vi "Edited-PumpCMD&Query(SubVI).vi"(0 "VISA资源名称":refnum<visa-resource-name>, 1 "允许执行时间":u32, 5 "命令":string, 7 "急停":string, 9 "查询":string, 11 "错误输入（无错误）":errorcluster, 12 "emergence":refnum<vi>) -> (4 "VISA资源名称输出":refnum<visa-resource-name>, 6 "Input string":string, 15 "错误输出":errorcluster)   [LabVIEW 2023]
uses:
  <vilib>/Instr/_visa.llb/VISA Flush IO Buffer Mask.ctl
panel:
  out "read buffer":string
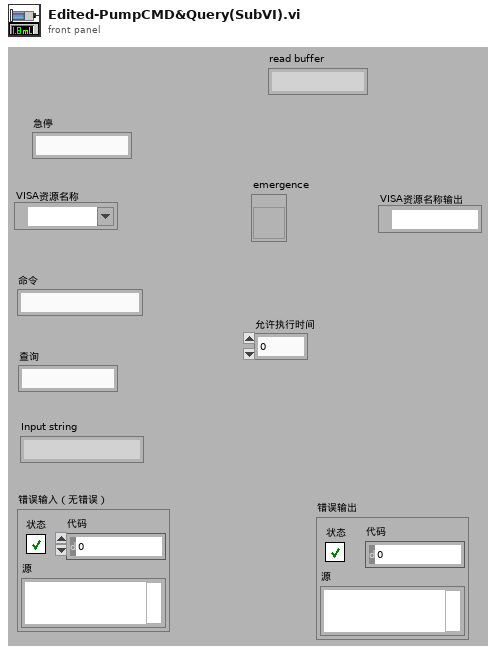
[diagram p1: front panel]
types:
  T1 = typedef "VISA Flush IO Buffer Mask.ctl" = u16
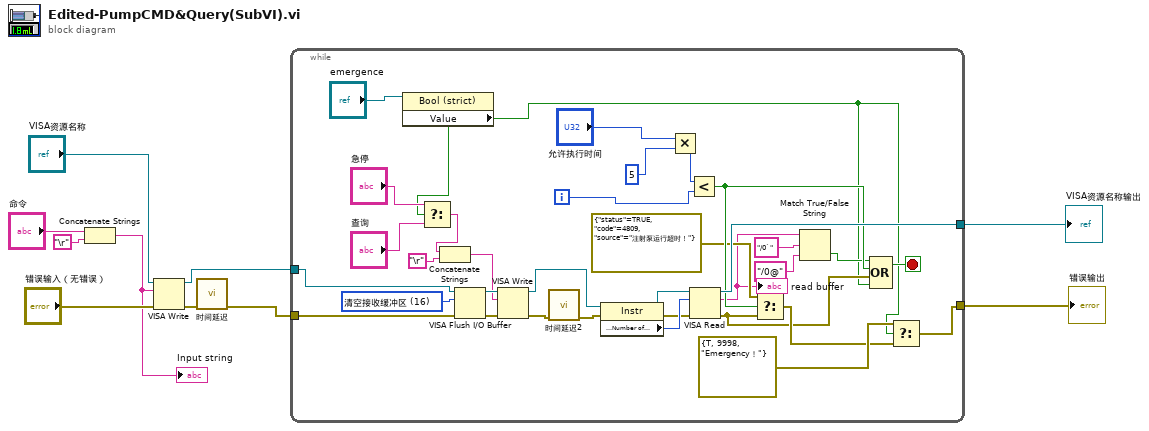
[diagram p0: block diagram]
diagram:
  n1 = Concatenate Strings("命令", "\r") -> (w4:string)
  "Input string" <- w4
  n2 = VISA Write(VISA resource name="VISA资源名称", write buffer=w4, error in (no error)="错误输入（无错误）") -> (VISA resource name out=w3:refnum<visa-resource-name>, error out=w1:errorcluster)  [unwired: 1 out]
  n3 = call "时间延迟"("error in (no error)"=w1) -> ("error out"=w2:errorcluster)  [unwired: 10 in]
  n4 = while {
    tunnel: w3 -> [w41]
    tunnel: w2 -> [w37]
    tunnel: [w43] -> w8
    tunnel: [w14] -> w7
    i -> [w20]
    stop <- w36 stop-if-true
    w39 = T1 16 items=["清空接收缓冲区"=16, "向设备写入传输缓冲区"=32, "清空接收缓冲区（无I/O）"=64, "清空传输缓冲区"=128] ("Mask")
    n5 = property class="Bool (strict)"(reference="emergence") -> ("Value"=w11:bool)  [unwired: 1 in, 2 out]
    n6 = Select(t="急停", s=w11, f="查询") -> (s? t:f=w16:string)
    n7 = Concatenate Strings(w16, "\r") -> (w32:string)
    n8 = VISA Flush I/O Buffer(VISA resource name=w41, mask (16)=w39, error in (no error)=w37) -> (VISA resource name out=w40:refnum<visa-resource-name>, error out=w38:errorcluster)
    n9 = VISA Write(VISA resource name=w40, write buffer=w32, error in (no error)=w38) -> (VISA resource name out=w44:refnum<visa-resource-name>, error out=w26:errorcluster)  [unwired: 1 out]
    n10 = call "时间延迟2"("error in (no error)"=w26) -> ("error out"=w25:errorcluster)  [unwired: 10 in]
    n11 = property class="Instr"(reference=w44, error in=w25) -> (reference out=w24:refnum<visa-resource-name>, error out=w27:errorcluster, "Serial Settings:Number of Bytes at Serial Port"=w42:u32)
    n12 = Multiply(x="允许执行时间", y=5 ("x")) -> (x*y=w21:u32)
    n13 = Less?(x=w21, y=w20) -> (x < y?=w35:bool)
    n14 = VISA Read(VISA resource name=w24, byte count=w42, error in (no error)=w27) -> (VISA resource name out=w43:refnum<visa-resource-name>, read buffer=w29:string, error out=w12:errorcluster)  [unwired: 1 out]
    "read buffer" <- w29
    n15 = Select(t=errorcluster {"status"=TRUE, "code"=4809, "source"="注射泵运行超时！"}, s=w35, f=w12) -> (s? t:f=w13:errorcluster)
    n16 = Match True/False String(2:"/0@" ("格式字符串"), 3:"/0`" ("格式字符串"), 4:w29) -> (0:w28:bool)  [unwired: 1 out]
    n17 = Compound Arithmetic op=OR(w28, w35, w12, w11) -> (w36:bool)
    n18 = Select(t=errorcluster {"status"=TRUE, "code"=9998, "source"="Emergency！"} ("error constant"), s=w11, f=w13) -> (s? t:f=w14:errorcluster)
  }
  "VISA资源名称输出" <- w8
  "错误输出" <- w7
